vi "Axsun module.vi"(7 "Action":T2=enum."Clock delay", 8 "error in (no error)":errorcluster, 10 "Clock delay":dbl) -> (0 "error out":errorcluster, 2 "output cluster":T1)   [LabVIEW 2018]
uses:
  Axsun action.ctl
  cluster_Axsun.ctl
  C:/Project/SerialSectionOCT/SerialSectOCT/Labview Software/Hardware Mfg/Axsun Laser/AxsunOCTControl.dll
  AxsunOCTControl.dll
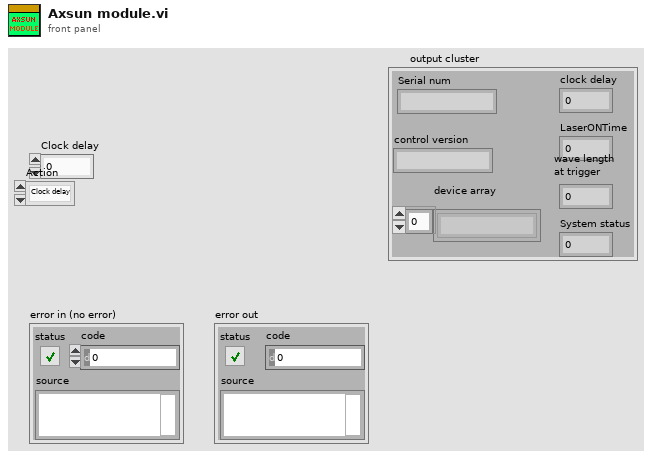
[diagram p1: front panel]
types:
  T1 = typedef "cluster_Axsun.ctl" = cluster{"device array":string[], "control version":string, "Serial num":string, "LaserONTime":i32, "wave length\nat trigger":dbl, "System status":dbl, "clock delay":u32}
  T2 = typedef "Axsun action.ctl" = enum16{"GetSystemStatus", "Clock delay", "GetLaserOnTime", "GetWaveLengthAtSweptTrigger", "Source current ON", "GetSerialNum", "GetControlVersion", "Laser ON", "Laser OFF", "Source current OFF", "Get laser handle", "Start Network Control Interface", "stop", "Create handle"}
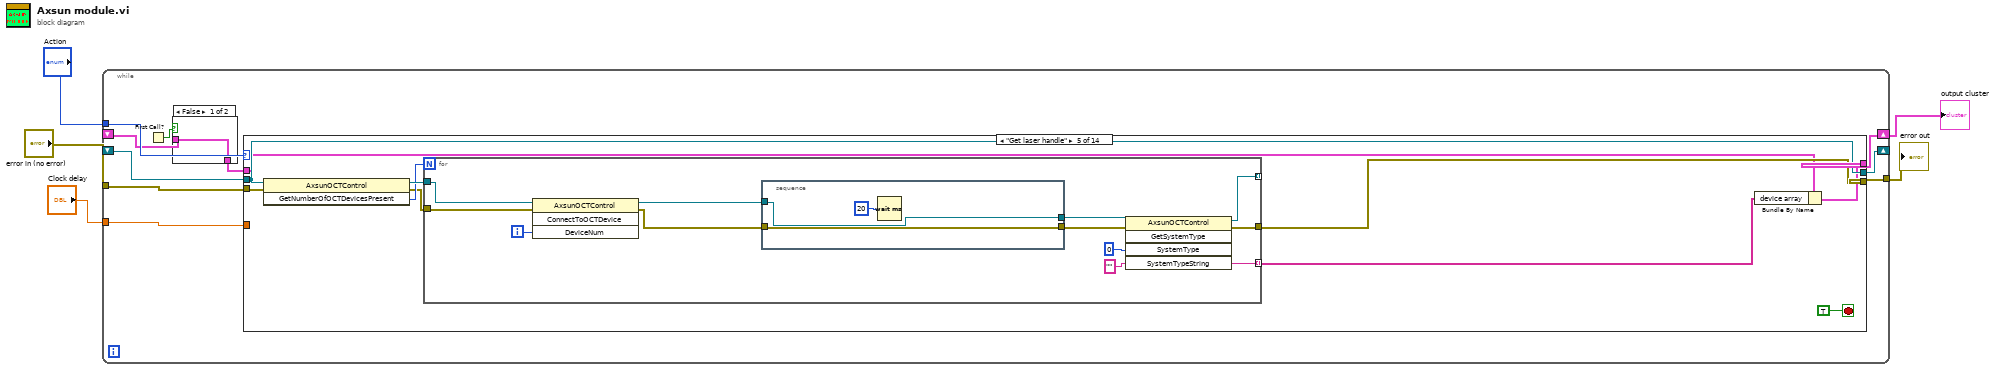
[diagram p0: block diagram]
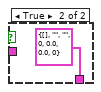
[diagram p2: hidden frame]
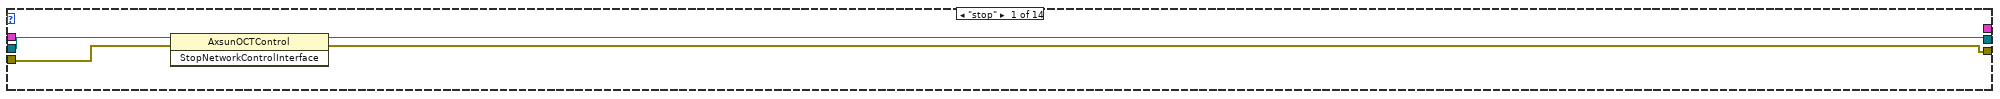
[diagram p3: hidden frame]
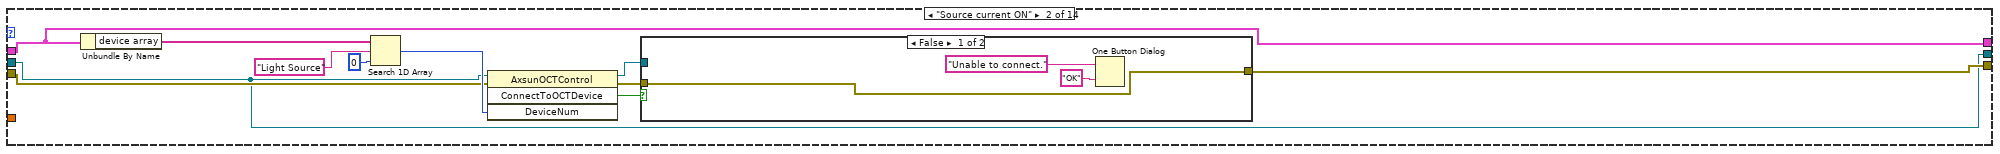
[diagram p4: hidden frame]
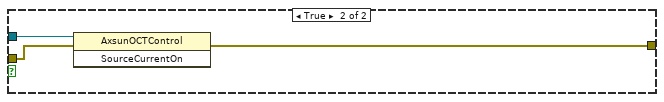
[diagram p5: hidden frame]
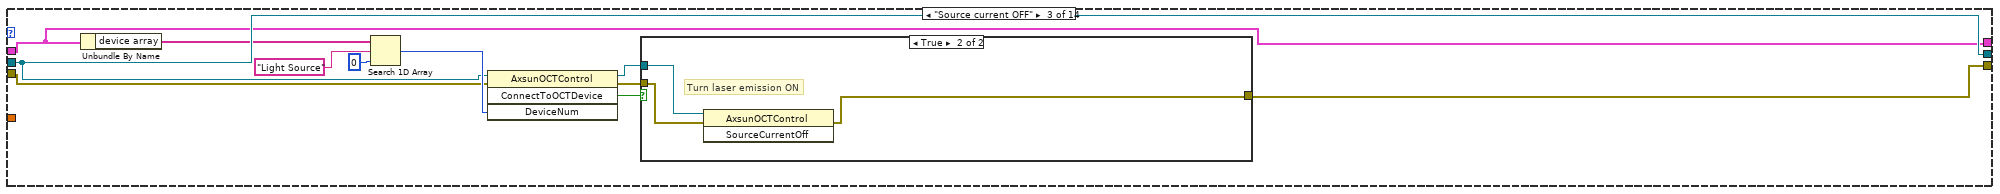
[diagram p6: hidden frame]
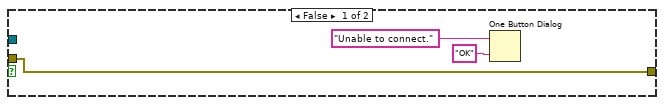
[diagram p7: hidden frame]
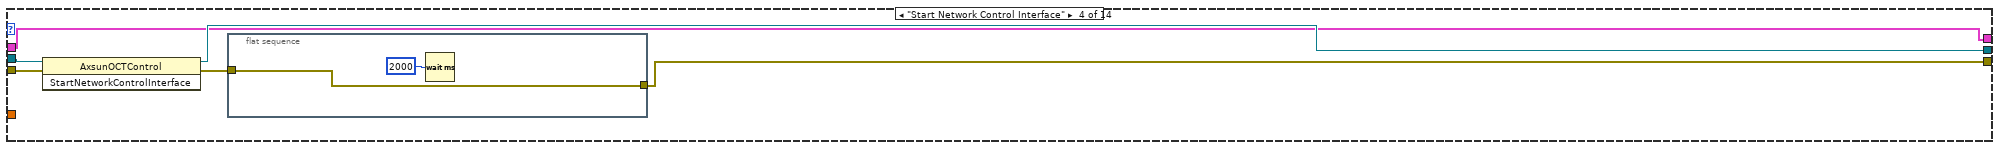
[diagram p8: hidden frame]
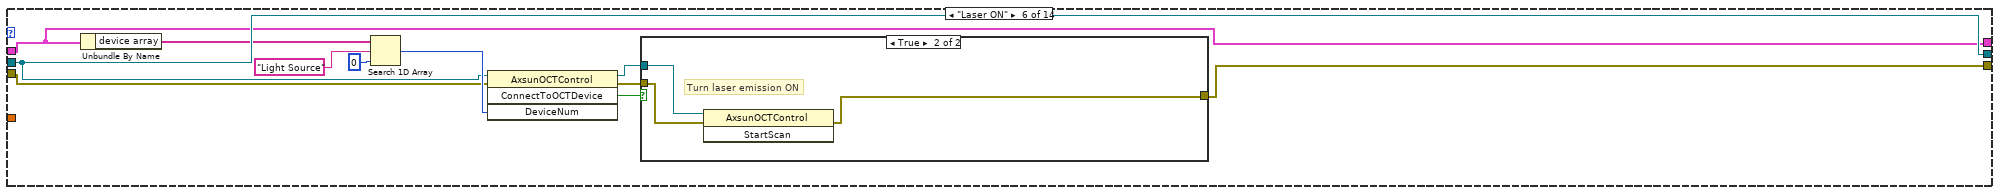
[diagram p9: hidden frame]
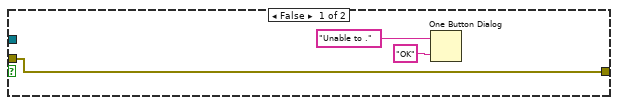
[diagram p10: hidden frame]
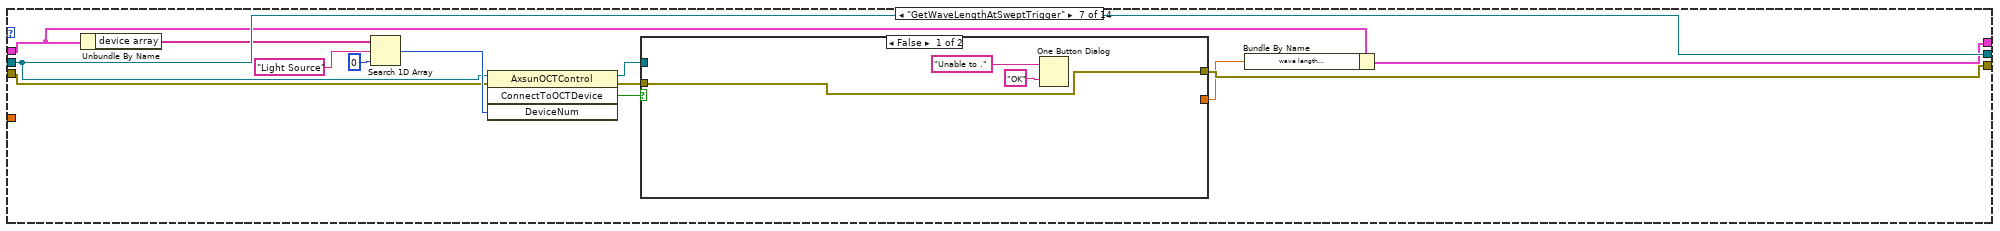
[diagram p11: hidden frame]
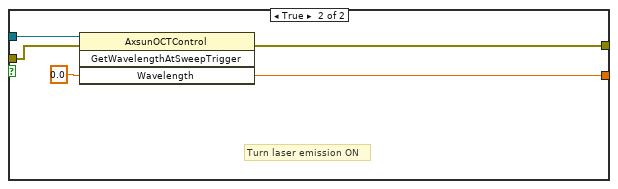
[diagram p12: hidden frame]
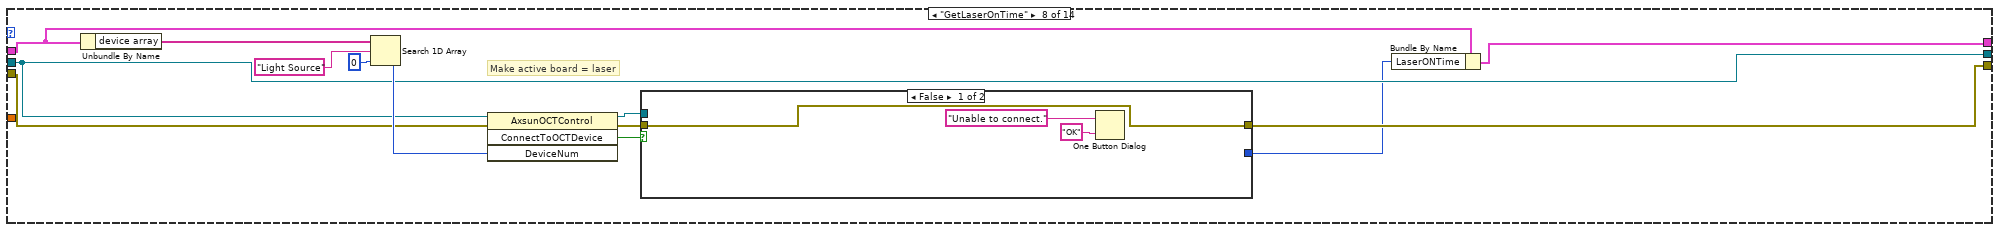
[diagram p13: hidden frame]
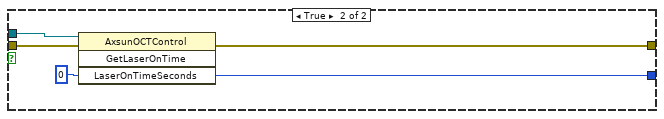
[diagram p14: hidden frame]
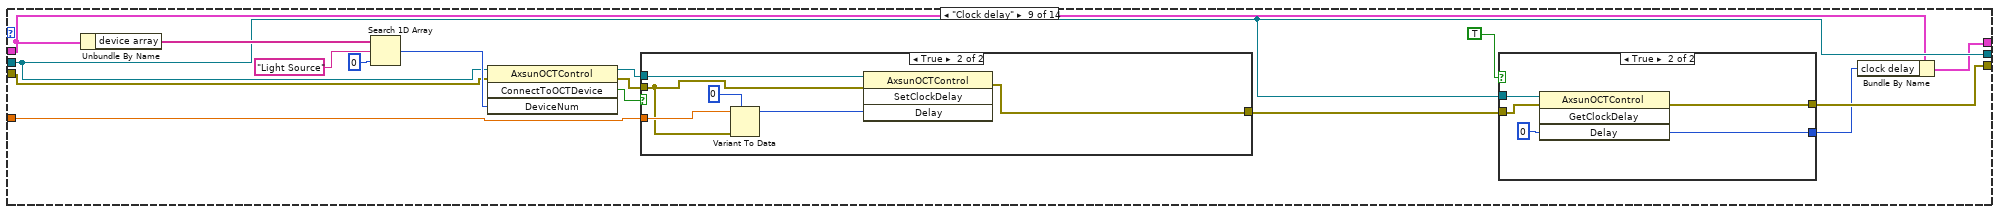
[diagram p15: hidden frame]
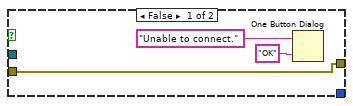
[diagram p16: hidden frame]
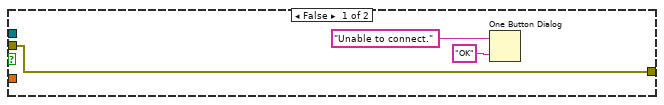
[diagram p17: hidden frame]
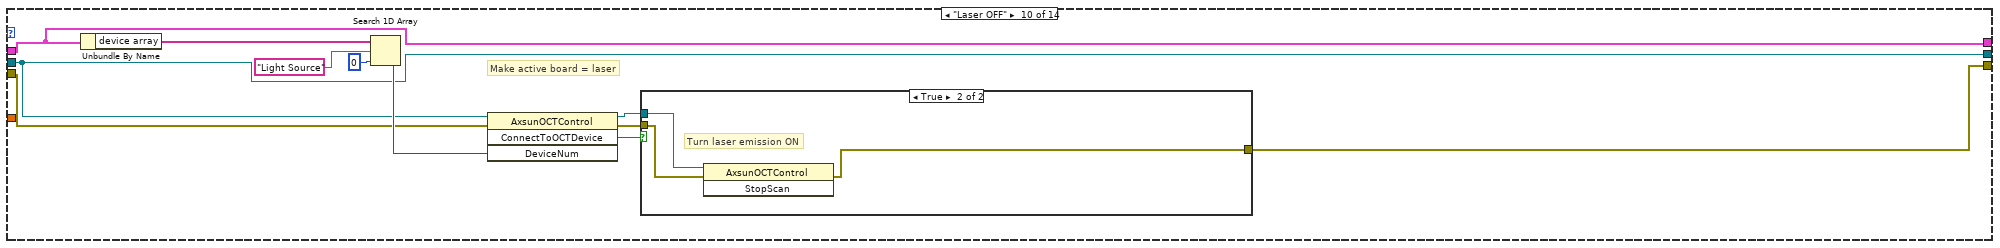
[diagram p18: hidden frame]
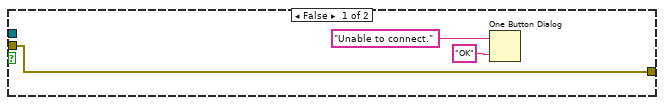
[diagram p19: hidden frame]
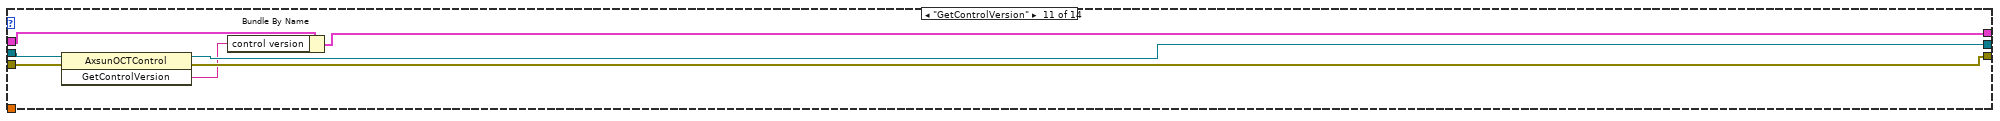
[diagram p20: hidden frame]
diagram:
  n1 = while {
    shift-right: [w15] -> _
    shift-left: _ -> [w14]
    tunnel: "error in (no error)" -> [w16]
    shift-right: [w12] -> w1
    shift-left: _ -> [w6]
    tunnel: [w13] -> w3
    tunnel: "Action" -> [w11]
    tunnel: "Clock delay" -> [w10]
    stop <- TRUE stop-if-true
    n2 = First Call?() -> (First Call?: T/F=w8:bool)
    n3 = case shown="False" w8 {
      tunnel: [w17 T1 {"device array"=[], "control version"="", "Serial num"="", "LaserONTime"=0, "wave length\nat trigger"=0.0, "System status"=0.0, "clock delay"=0} ("output cluster")] -> w7
      tunnel: w6 -> [w17 _]
      frame False {
      }
      frame True {
      }
    }
    n4 = case shown="\"Get laser handle\"" w11 {
      tunnel: w16 -> [w21 w27 w43 w61 w73 w93 w111 w133 w156 w185 w203 w210 w232 _]
      tunnel: [w20 w25 w42 w58 w68 w91 w112 w131 w153 w183 w201 w211 w226 w250] -> w15
      tunnel: w14 -> [w22 w25 w42 w62 w68 w91 w112 w131 w153 w183 w204 w211 w233 _]
      tunnel: [w19 w26 w44 w59 w69 w92 w110 w132 w152 w184 w202 w209 w231 w249] -> w13
      tunnel: [_ w24 w41 w57 w67 w90 w107 w128 w150 w182 w199 w205 w227 w248] -> w12
      tunnel: w7 -> [_ w24 w41 w57 w65 w90 w108 w129 w151 w182 w200 w207 w229 w248]
      tunnel: w10 -> [_ _ _ _ _ _ _ _ w148 _ _ _ _ _]
      frame "stop" {
        n5 = invoke class="AxsunOCTControl" method="StopNetworkControlInterface"(reference=w22, error in=w21) -> (reference out=w20:refnum<k24>, error out=w19:errorcluster)  [unwired: 1 in, 1 out]
      }
      frame "Source current ON" {
        n6 = Unbundle By Name(w24) -> ("device array"=w23:string[])
        n7 = Search 1D Array(1D array=w23, element="Light Source", start index (0)=0) -> (index of element=w31:i32)
        n8 = invoke class="AxsunOCTControl" method="ConnectToOCTDevice"(reference=w25, error in=w27, "DeviceNum"=w31) -> (reference out=w30:refnum<k24>, error out=w29:errorcluster, "ConnectToOCTDevice"=w28:bool)  [unwired: 1 in, 1 out]
        n9 = case shown="False" w28 {
          tunnel: w30 -> [_ w39]
          tunnel: w29 -> [w36 w38]
          tunnel: [w36 w37] -> w26
          frame False {
            n10 = One Button Dialog(message="Unable to connect.", button name ("OK")="OK") -> ()  [unwired: 1 out]
          }
          frame True {
            n11 = invoke class="AxsunOCTControl" method="SourceCurrentOn"(reference=w39, error in=w38) -> (error out=w37:errorcluster)  [unwired: 1 in, 2 out]
          }
        }
      }
      frame "Source current OFF" {
        n12 = Unbundle By Name(w41) -> ("device array"=w40:string[])
        n13 = Search 1D Array(1D array=w40, element="Light Source", start index (0)=0) -> (index of element=w48:i32)
        n14 = invoke class="AxsunOCTControl" method="ConnectToOCTDevice"(reference=w42, error in=w43, "DeviceNum"=w48) -> (reference out=w47:refnum<k24>, error out=w46:errorcluster, "ConnectToOCTDevice"=w45:bool)  [unwired: 1 in, 1 out]
        n15 = case shown="True" w45 {
          tunnel: w47 -> [_ w56]
          tunnel: w46 -> [w53 w55]
          tunnel: [w53 w54] -> w44
          frame False {
            n16 = One Button Dialog(message="Unable to connect.", button name ("OK")="OK") -> ()  [unwired: 1 out]
          }
          frame True {
            # "Turn laser emission ON"
            n17 = invoke class="AxsunOCTControl" method="SourceCurrentOff"(reference=w56, error in=w55) -> (error out=w54:errorcluster)  [unwired: 1 in, 2 out]
          }
        }
      }
      frame "Start Network Control Interface" {
        n18 = invoke class="AxsunOCTControl" method="StartNetworkControlInterface"(reference=w62, error in=w61) -> (reference out=w58:refnum<k24>, error out=w60:errorcluster)  [unwired: 1 in, 1 out]
        n19 = flat-sequence {
          tunnel: w60 -> [w63]
          tunnel: [w63] -> w59
          frame #0 {
            n20 = Wait (ms)(milliseconds to wait=2000) -> ()  [unwired: 1 out]
          }
        }
      }
      frame "Get laser handle" {
        n21 = invoke class="AxsunOCTControl" method="GetNumberOfOCTDevicesPresent"(reference=w68, error in=w73) -> (reference out=w72:refnum<k24>, error out=w70:errorcluster, "GetNumberOfOCTDevicesPresent"=w71:i32)  [unwired: 1 in]
        n22 = for {
          N: w71 -> [_]
          tunnel: w72 -> [w79]
          tunnel: w70 -> [w78]
          tunnel: [w74] -> w66 mode=indexing
          tunnel: [w76] -> w69
          tunnel: [w75] -> _ mode=indexing
          i -> [w77]
          n23 = invoke class="AxsunOCTControl" method="ConnectToOCTDevice"(reference=w79, error in=w78, "DeviceNum"=w77) -> (reference out=w83:refnum<k24>, error out=w82:errorcluster)  [unwired: 1 in, 2 out]
          n24 = stacked-sequence {
            tunnel: w83 -> [w88]
            tunnel: [w88] -> w81
            tunnel: w82 -> [w87]
            tunnel: [w87] -> w80
            frame #0 {
              n25 = Wait (ms)(milliseconds to wait=u32 20) -> ()  [unwired: 1 out]
            }
          }
          n26 = invoke class="AxsunOCTControl" method="GetSystemType"(reference=w81, error in=w80, "SystemType"=u32 0, "SystemTypeString"="") -> (reference out=w75:refnum<k24>, error out=w76:errorcluster, "SystemTypeString"=w74:string)  [unwired: 1 in, 2 out]
        }
        n27 = Bundle By Name(cluster=w65, "device array"=w66) -> (w67:T1)
      }
      frame "Laser ON" {
        n28 = Unbundle By Name(w90) -> ("device array"=w89:string[])
        n29 = Search 1D Array(1D array=w89, element="Light Source", start index (0)=0) -> (index of element=w97:i32)
        n30 = invoke class="AxsunOCTControl" method="ConnectToOCTDevice"(reference=w91, error in=w93, "DeviceNum"=w97) -> (reference out=w96:refnum<k24>, error out=w95:errorcluster, "ConnectToOCTDevice"=w94:bool)  [unwired: 1 in, 1 out]
        n31 = case shown="True" w94 {
          tunnel: w96 -> [_ w105]
          tunnel: w95 -> [w102 w104]
          tunnel: [w102 w103] -> w92
          frame False {
            n32 = One Button Dialog(message="Unable to .", button name ("OK")="OK") -> ()  [unwired: 1 out]
          }
          frame True {
            # "Turn laser emission ON"
            n33 = invoke class="AxsunOCTControl" method="StartScan"(reference=w105, error in=w104) -> (error out=w103:errorcluster)  [unwired: 1 in, 2 out]
          }
        }
      }
      frame "GetWaveLengthAtSweptTrigger" {
        n34 = Unbundle By Name(w108) -> ("device array"=w109:string[])
        n35 = Search 1D Array(1D array=w109, element="Light Source", start index (0)=0) -> (index of element=w116:i32)
        n36 = invoke class="AxsunOCTControl" method="ConnectToOCTDevice"(reference=w112, error in=w111, "DeviceNum"=w116) -> (reference out=w115:refnum<k24>, error out=w114:errorcluster, "ConnectToOCTDevice"=w113:bool)  [unwired: 1 in, 1 out]
        n37 = case shown="False" w113 {
          tunnel: w115 -> [_ w126]
          tunnel: w114 -> [w121 w125]
          tunnel: [w121 w124] -> w110
          tunnel: [_ w122] -> w106
          frame False {
            n38 = One Button Dialog(message="Unable to .", button name ("OK")="OK") -> ()  [unwired: 1 out]
          }
          frame True {
            # "Turn laser emission ON"
            n39 = invoke class="AxsunOCTControl" method="GetWavelengthAtSweepTrigger"(reference=w126, error in=w125, "Wavelength"=0.0) -> (error out=w124:errorcluster, "Wavelength"=w122:dbl)  [unwired: 1 in, 2 out]
          }
        }
        n40 = Bundle By Name(cluster=w108, "wave length\nat trigger"=w106) -> (w107:T1)
      }
      frame "GetLaserOnTime" {
        # "Make active board = laser"
        n41 = Unbundle By Name(w129) -> ("device array"=w130:string[])
        n42 = Search 1D Array(1D array=w130, element="Light Source", start index (0)=0) -> (index of element=w139:i32)
        n43 = invoke class="AxsunOCTControl" method="ConnectToOCTDevice"(reference=w131, error in=w133, "DeviceNum"=w139) -> (reference out=w135:refnum<k24>, error out=w136:errorcluster, "ConnectToOCTDevice"=w134:bool)  [unwired: 1 in, 1 out]
        n44 = case shown="False" w134 {
          tunnel: w136 -> [w142 w146]
          tunnel: w135 -> [_ w147]
          tunnel: [w142 w145] -> w132
          tunnel: [_ w143] -> w127
          frame False {
            n45 = One Button Dialog(message="Unable to connect.", button name ("OK")="OK") -> ()  [unwired: 1 out]
          }
          frame True {
            n46 = invoke class="AxsunOCTControl" method="GetLaserOnTime"(reference=w147, error in=w146, "LaserOnTimeSeconds"=u32 0) -> (error out=w145:errorcluster, "LaserOnTimeSeconds"=w143:u32)  [unwired: 1 in, 2 out]
          }
        }
        n47 = Bundle By Name(cluster=w129, "LaserONTime"=w127) -> (w128:T1)
      }
      frame "Clock delay" {
        n48 = Unbundle By Name(w151) -> ("device array"=w157:string[])
        n49 = Search 1D Array(1D array=w157, element="Light Source", start index (0)=0) -> (index of element=w161:i32)
        n50 = invoke class="AxsunOCTControl" method="ConnectToOCTDevice"(reference=w153, error in=w156, "DeviceNum"=w161) -> (reference out=w160:refnum<k24>, error out=w159:errorcluster, "ConnectToOCTDevice"=w158:bool)  [unwired: 1 in, 1 out]
        n51 = case shown="True" w158 {
          tunnel: w160 -> [_ w180]
          tunnel: w159 -> [w174 w176]
          tunnel: [w174 w175] -> w155
          tunnel: w148 -> [_ w179]
          frame False {
            n52 = One Button Dialog(message="Unable to connect.", button name ("OK")="OK") -> ()  [unwired: 1 out]
          }
          frame True {
            n53 = Variant To Data(error in=w176, type=u32 0 ("Delay"), Variant=w179) -> (data=w177:u32)  [unwired: 1 out]
            n54 = invoke class="AxsunOCTControl" method="SetClockDelay"(reference=w180, error in=w176, "Delay"=w177) -> (error out=w175:errorcluster)  [unwired: 1 in, 3 out]
          }
        }
        n55 = case shown="True" TRUE {
          tunnel: w155 -> [w166 w170]
          tunnel: w153 -> [_ w171]
          tunnel: [w166 w169] -> w152
          tunnel: [_ w167] -> w149
          frame False {
            n56 = One Button Dialog(message="Unable to connect.", button name ("OK")="OK") -> ()  [unwired: 1 out]
          }
          frame True {
            n57 = invoke class="AxsunOCTControl" method="GetClockDelay"(reference=w171, error in=w170, "Delay"=u32 0) -> (error out=w169:errorcluster, "Delay"=w167:u32)  [unwired: 1 in, 2 out]
          }
        }
        n58 = Bundle By Name(cluster=w151, "clock delay"=w149) -> (w150:T1)
      }
      frame "Laser OFF" {
        # "Make active board = laser"
        n59 = Unbundle By Name(w182) -> ("device array"=w181:string[])
        n60 = Search 1D Array(1D array=w181, element="Light Source", start index (0)=0) -> (index of element=w189:i32)
        n61 = invoke class="AxsunOCTControl" method="ConnectToOCTDevice"(reference=w183, error in=w185, "DeviceNum"=w189) -> (reference out=w188:refnum<k24>, error out=w187:errorcluster, "ConnectToOCTDevice"=w186:bool)  [unwired: 1 in, 1 out]
        n62 = case shown="True" w186 {
          tunnel: w188 -> [_ w197]
          tunnel: w187 -> [w194 w196]
          tunnel: [w194 w195] -> w184
          frame False {
            n63 = One Button Dialog(message="Unable to connect.", button name ("OK")="OK") -> ()  [unwired: 1 out]
          }
          frame True {
            # "Turn laser emission ON"
            n64 = invoke class="AxsunOCTControl" method="StopScan"(reference=w197, error in=w196) -> (error out=w195:errorcluster)  [unwired: 1 in, 2 out]
          }
        }
      }
      frame "GetControlVersion" {
        n65 = invoke class="AxsunOCTControl" method="GetControlVersion"(reference=w204, error in=w203) -> (reference out=w201:refnum<k24>, error out=w202:errorcluster, "GetControlVersion"=w198:string)  [unwired: 1 in]
        n66 = Bundle By Name(cluster=w200, "control version"=w198) -> (w199:T1)
      }
      frame "GetSerialNum" {
        n67 = Unbundle By Name(w207) -> ("device array"=w208:string[])
        n68 = Search 1D Array(1D array=w208, element="Light Source", start index (0)=0) -> (index of element=w215:i32)
        n69 = invoke class="AxsunOCTControl" method="ConnectToOCTDevice"(reference=w211, error in=w210, "DeviceNum"=w215) -> (reference out=w214:refnum<k24>, error out=w213:errorcluster, "ConnectToOCTDevice"=w212:bool)  [unwired: 1 in, 1 out]
        n70 = case shown="True" w212 {
          tunnel: w214 -> [_ w225]
          tunnel: w213 -> [w220 w224]
          tunnel: [w220 w223] -> w209
          tunnel: [_ w221] -> w206
          frame False {
            n71 = One Button Dialog(message="Unable to connect.", button name ("OK")="OK") -> ()  [unwired: 1 out]
          }
          frame True {
            n72 = invoke class="AxsunOCTControl" method="GetSerialNum"(reference=w225, error in=w224, "SerialNum"="") -> (error out=w223:errorcluster, "SerialNum"=w221:string)  [unwired: 1 in, 2 out]
          }
        }
        n73 = Bundle By Name(cluster=w207, "Serial num"=w206) -> (w205:T1)
      }
      frame "GetSystemStatus" {
        # "Make active board = laser"
        n74 = Unbundle By Name(w229) -> ("device array"=w230:string[])
        n75 = Search 1D Array(1D array=w230, element="Light Source", start index (0)=0) -> (index of element=w238:i32)
        n76 = invoke class="AxsunOCTControl" method="ConnectToOCTDevice"(reference=w233, error in=w232, "DeviceNum"=w238) -> (reference out=w226:refnum<k24>, error out=w234:errorcluster, "ConnectToOCTDevice"=w235:bool)  [unwired: 1 in, 1 out]
        n77 = case shown="True" w235 {
          tunnel: w234 -> [w241 w246]
          tunnel: w226 -> [_ w247]
          tunnel: [w241 w243] -> w231
          tunnel: [_ w242] -> w228
          frame False {
            n78 = One Button Dialog(message="Unable to connect.", button name ("OK")="OK") -> ()  [unwired: 1 out]
          }
          frame True {
            n79 = invoke class="AxsunOCTControl" method="GetSystemStatus"(reference=w247, error in=w246, "StatusArray"=u32[] [], "StatusWordsReturned"=u32 0) -> (error out=w243:errorcluster, "StatusWordsReturned"=w242:u32)  [unwired: 1 in, 3 out]
          }
        }
        n80 = Bundle By Name(cluster=w229, "System status"=w228) -> (w227:T1)
      }
      frame "Create handle" {
        n81 = constructor class="AxsunOCTControl"() -> (reference out=w250:refnum<k24>, error out=w249:errorcluster)  [unwired: 3 in, 1 out]
      }
    }
  }
  "error out" <- w3
  "output cluster" <- w1
